vi "Midi_write multiple....vi"(8 "error in (no error)":errorcluster, 10 "console in":string, 11 "to write":string) -> (0 "error out":errorcluster, 2 "console out":string)   [LabVIEW 2022 SP3]
panel:
  out "string array":string[](array[string])
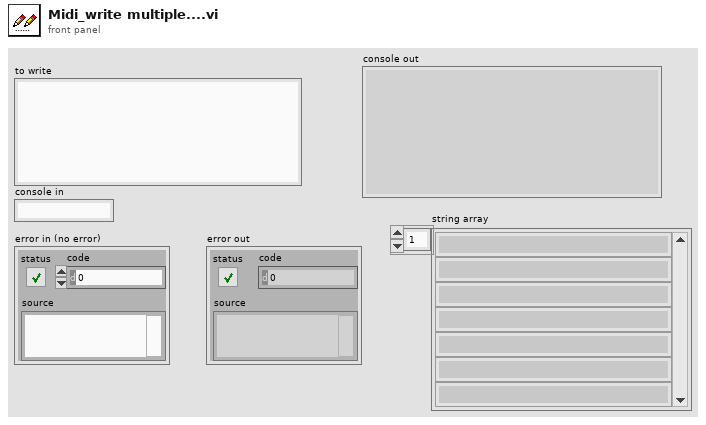
[diagram p1: front panel]
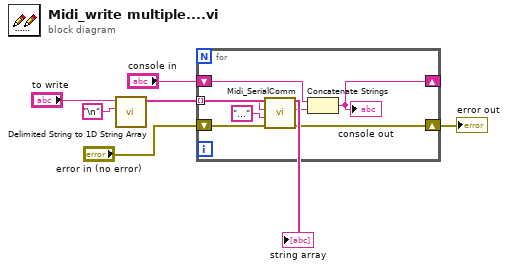
[diagram p0: block diagram]
diagram:
  n1 = call <vilib>:"Delimited String to 1D String Array.vi"("delimiter"="\n" ("delimiter (Tab)"), "delimited string"="to write") -> ("string array"=w1:string[])  [unwired: 9 in]
  "string array" <- w1
  n2 = for {
    shift-right: [w10] -> w4
    shift-left: "error in (no error)" -> [w13]
    shift-right: [w7] -> _
    shift-left: "console in" -> [w11]
    tunnel: w1 -> [w8] mode=indexing
    n3 = call "Midi_SerialComm.vi"("error in (no error)"=w13, "wait for"="...", "To send"=w8) -> ("error out"=w10:errorcluster, "read"=w12:string)  [unwired: 7 in]
    n4 = Concatenate Strings(w11, w12) -> (w7:string)
    "console out" <- w7
  }
  "error out" <- w4
